vi "load file to imaq image v2.vi"(8 "error in (no error)":errorcluster, 10 "Image Name":string="untitledCOLOR", 11 "path to BMP file":path=path "C:/Andy/FRC/FRC 2017/Fall PreSeason Exercise/valve image.bmp") -> (0 "error out":errorcluster, 3 "Image":T1(plugin-control))   [LabVIEW 2016]
uses:
  <vilib>/vision/NI_Vision_Development_Module.lvlib
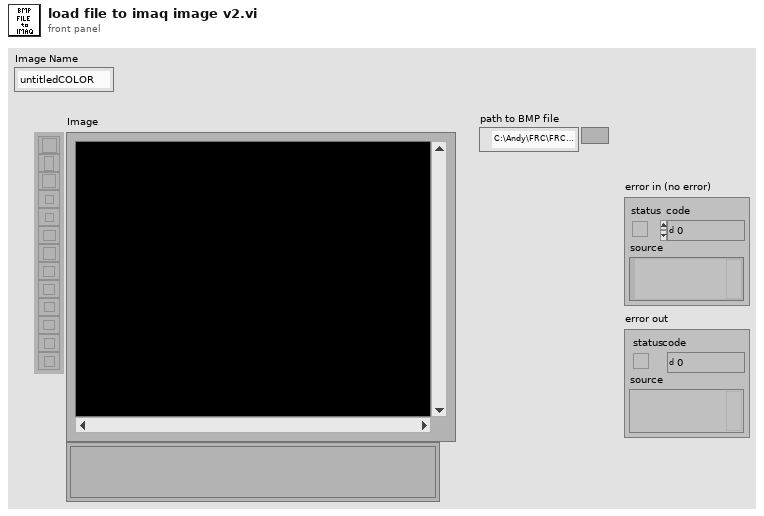
[diagram p1: front panel]
types:
  T1 = typedef "IMAQ Image.ctl" = refnum<image>
  T2 = typedef "Image Type" = u32
  T3 = typedef "imagedata.ctl" = cluster{"image type":i32, "image depth":i32, "image":u8[], "mask":u8[], "colors":u32[], "Rectangle":cluster{"left":i16, "top":i16, "right":i16, "bottom":i16}}
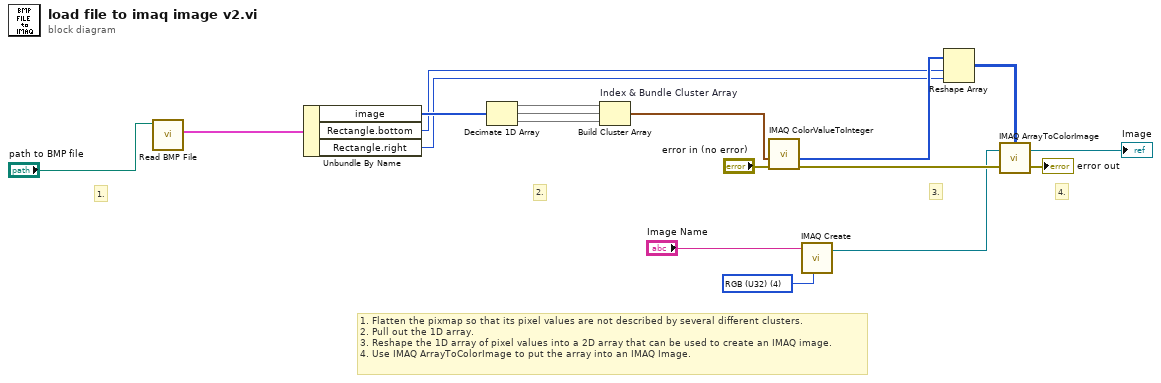
[diagram p0: block diagram]
diagram:
  w4 = T2 4 items=["Grayscale (U8)", "Grayscale (I16)", "Grayscale (SGL)", "Complex (CSG)", "RGB (U32)", "HSL (U32)", "RGB (U64)", "Grayscale (U16)"] ("Image Type")
  # "1. Flatten the pixmap so that its pixel values are not described by several different clusters.\n2. Pull out the 1D array.\n3. Reshape the 1D array of pixel values into a 2D array that can be used to create an IMAQ image.\n4. Use IMAQ ArrayToColorImage to put the array into an IMAQ Image."
  # "4."
  # "3."
  # "2."
  # "1."
  n1 = call <vilib>:"Read BMP File.vi"("path to BMP file"="path to BMP file") -> ("image data"=w1:T3)  [unwired: 8 in, 2 out]
  n2 = Unbundle By Name "Unbundle By Name"(w1) -> ("image"=w18:u8[], "Rectangle.bottom"=w12:i16, "Rectangle.right"=w11:i16)
  n3 = Decimate 1D Array "Decimate 1D Array"(w18) -> (w17:u8[], w16:u8[], w15:u8[])
  n4 = Build Cluster Array "Index & Bundle Cluster Array"(w17, w16, w15) -> (w14:cluster{u8, u8, u8}[])
  n5 = call "IMAQ ColorValueToInteger"("error in (no error)"="error in (no error)", "1D Color value array"=w14) -> ("1D U32 array"=w13:u32[], "error out"=w8:errorcluster)  [unwired: 3 in, 2 out]
  n6 = call "IMAQ Create"("Image Name"="Image Name", "Image Type"=w4) -> ("New Image"=w2:T1)  [unwired: 3 in, 1 out]
  n7 = Reshape Array(w13, w12, w11) -> (w10:u32[][])
  n8 = call "IMAQ ArrayToColorImage"("Image Pixels (U32)"=w10, "Image"=w2, "error in (no error)"=w8) -> ("Image Out"=→"Image":T1, "error out"=→"error out":errorcluster)  [unwired: 2 in]
